vi "Handle Error.vi"(8 "error in (no error)":errorcluster, 11 "Measure Object in":refnum<class "Measure Object.lvclass">) -> (0 "error out":errorcluster, 2 "stop actor?":bool=TRUE, 3 "Measure Object out":refnum<class "Measure Object.lvclass">)   [LabVIEW 2016, in "Measure Object.lvclass"]
doc: "(<B>Filename</B>: Actor Framework.lvlib:Actor.lvclass:Handle Error.vi)\n\nDefines how the actor handles an error that occurred while processing a message. By default, this method does nothing except stop the actor."
uses:
  Measure Object.lvclass
  Measure Object.lvclass/Measure Object.ctl
  Read Name.vi
  <vilib>/Utility/error.llb/Error Cluster From Error Code.vi
  <vilib>/ActorFramework/Actor/Actor.lvclass
  <vilib>/ErrorRing/Error Ring.xnode
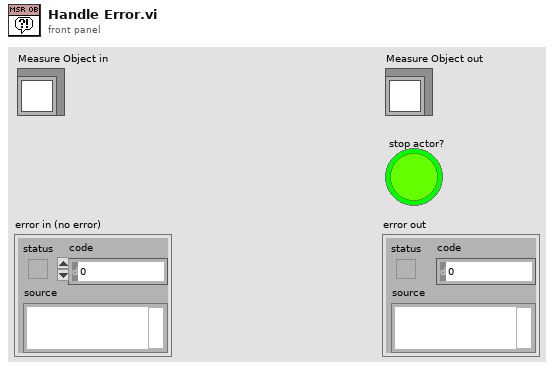
[diagram p1: front panel]
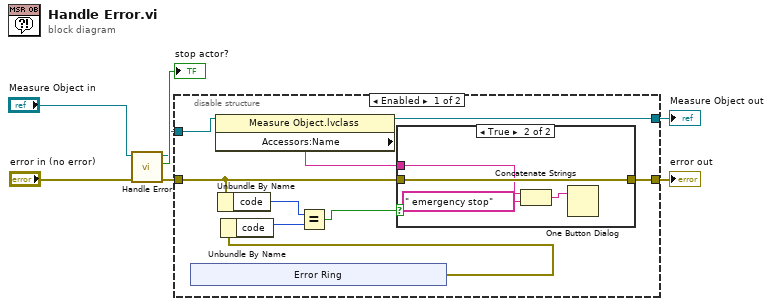
[diagram p0: block diagram]
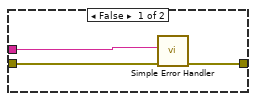
[diagram p2: hidden frame]
diagram:
  n1 = call-parent "Handle Error.vi"("error in (no error)"="error in (no error)", "Actor in"="Measure Object in") -> ("error out"=w4:errorcluster, "stop actor?"=→"stop actor?":bool, "Actor out"=w2:refnum<class "Measure Object.lvclass">)  [unwired: 7 in]
  n2 = disable-structure shown="Enabled" {
    disable-tunnel: w4 -> [w12 w29]
    disable-tunnel: [w16 w29] -> w3
    disable-tunnel: w2 -> [w15 w28]
    disable-tunnel: [w13 w28] -> w1
    frame Enabled {
      n3 = xnode "Error Ring"() -> ("error out"=w11:errorcluster)
      n4 = property class="Measure Object.lvclass"(reference=w15) -> (reference out=w13:refnum<class "Measure Object.lvclass">, "Accessors:Name"=w14:string)  [unwired: 1 in, 1 out]
      n5 = Unbundle By Name(w12) -> ("code"=w10:i32)
      n6 = Unbundle By Name(w11) -> ("code"=w9:i32)
      n7 = Equal?(x=w10, y=w9) -> (x = y?=w8:bool)
      n8 = case shown="True" w8 {
        tunnel: w12 -> [w23 w27]
        tunnel: [w22 w27] -> w16
        tunnel: w14 -> [w21 w26]
        frame False {
          n9 = call <vilib>:"Simple Error Handler.vi"("error source (\" \")"=w21, "error in (no error)"=w23) -> ("error out"=w22:errorcluster)  [unwired: 3 in, 4 out]
        }
        frame True {
          n10 = Concatenate Strings(w26, " emergency stop" ("string")) -> (w24:string)
          n11 = One Button Dialog(message=w24) -> ()  [unwired: 1 in, 1 out]
        }
      }
    }
    frame Disabled {
    }
  }
  "Measure Object out" <- w1
  "error out" <- w3
